vi "ApplicationStatusView.vi"(10 "Communicator":refnum<class "M1M3SAL.lvclass">, 11 "UserEvents":refnum<class "UserEvents.lvclass">) -> ()   [LabVIEW 2016, in "M1M3SupportViews.lvlib"]
uses:
  M1M3SupportViews.lvlib
  UserEvents/UserEvents.lvclass
  Communicator/M1M3SAL/M1M3SAL.lvclass
  DataTypes/Topics/Parts/SummaryStates.ctl
  DataTypes/Topics/Parts/DetailedStates.ctl
  UserEvents/UserEvents.lvclass/UserEvents.ctl
  DataTypes/Topics/M1M3SupportTopics.lvlib
panel:
  out "MinorRevision":u8[](array[numeric])
  out "MajorRevision":u8[](array[numeric])
  out "ReferencePosition":i32[](array[numeric])
  out "ILCUniqueId":i64[](array[numeric])
  out "SettingsApplied":string
  out "RecommendedSettingsVersion":string
  out "DetailedStates":T1
  out "ERxFrame":u32
  out "ETxFrame":u32
  out "FPGA Timestamp":dbl
  out "Timestamp":dbl
  out "SummaryStates":T2
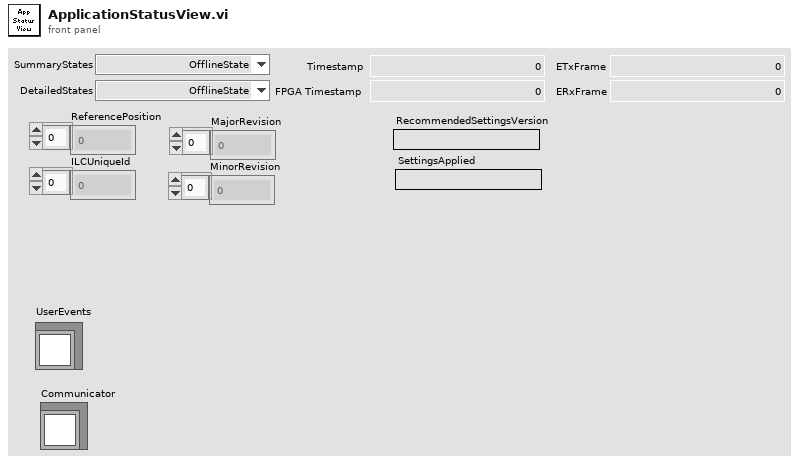
[diagram p1: front panel]
types:
  T1 = typedef "M1M3SupportTopics.lvlib/DetailedStates.ctl" = enum16{"OfflineState", "InitialState", "StandbyState", "DisabledState", "ParkedState", "FaultState", "ParkedMaintenanceState", "ActiveMaintenanceState"}
  T2 = typedef "M1M3SupportTopics.lvlib/SummaryStates.ctl" = enum16{"OfflineState", "StandbyState", "DisabledState", "EnabledState", "FaultState"}
  T3 = typedef "M1M3SupportTypes.lvlib/SummaryStates.ctl" = enum16{"OfflineState", "StandbyState", "DisabledState", "EnabledState", "FaultState"}
  T4 = typedef "M1M3SupportTopics.lvlib/Timestamp.ctl" = dbl
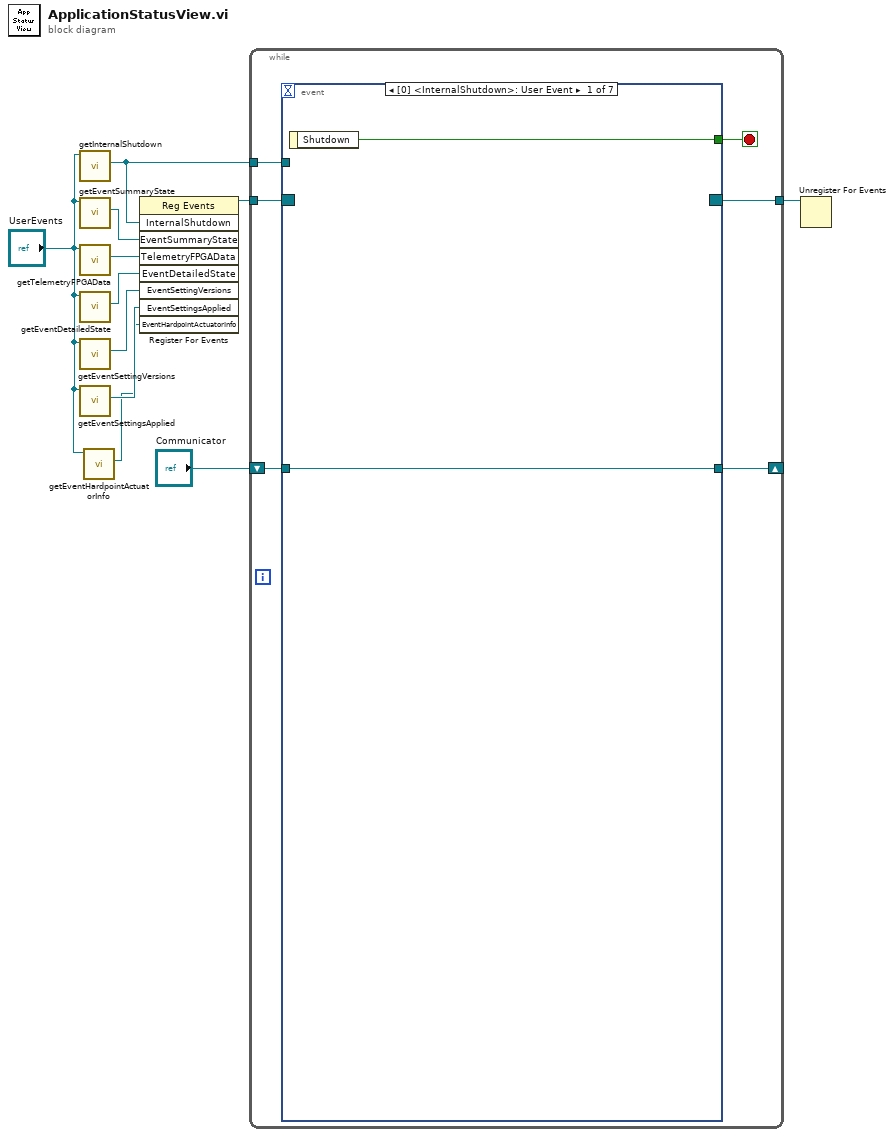
[diagram p0: block diagram]
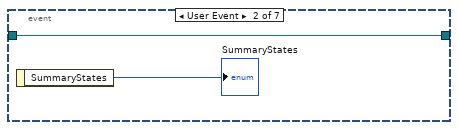
[diagram p2: hidden frame]
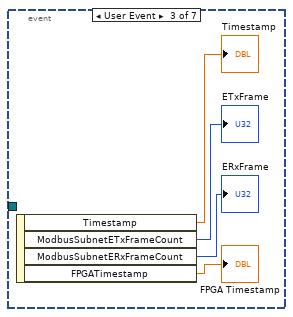
[diagram p3: hidden frame]
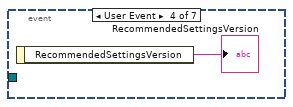
[diagram p4: hidden frame]
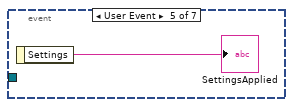
[diagram p5: hidden frame]
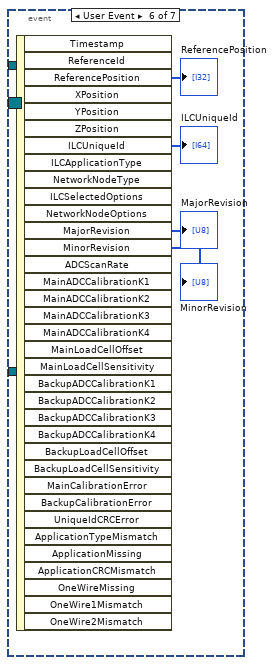
[diagram p6: hidden frame]
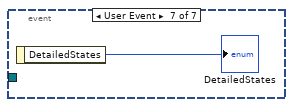
[diagram p7: hidden frame]
diagram:
  n1 = call "getInternalShutdown.vi"("UserEvents in"="UserEvents") -> ("InternalShutdown"=w7:refnum<user-event>)  [unwired: 9 in, 1 out]
  n2 = call "getEventSummaryState.vi"("UserEvents in"="UserEvents") -> ("EventSummaryState"=w11:refnum<user-event>)  [unwired: 9 in, 1 out]
  n3 = call "getTelemetryFPGAData.vi"("UserEvents in"="UserEvents") -> ("TelemetryFPGAData"=w6:refnum<user-event>)  [unwired: 9 in, 1 out]
  n4 = call "getEventDetailedState.vi"("UserEvents in"="UserEvents") -> ("EventDetailedState"=w5:refnum<user-event>)  [unwired: 9 in, 1 out]
  n5 = call "getEventSettingVersions.vi"("UserEvents in"="UserEvents") -> ("EventSettingVersions"=w4:refnum<user-event>)  [unwired: 9 in, 1 out]
  n6 = call "getEventSettingsApplied.vi"("UserEvents in"="UserEvents") -> ("EventSettingsApplied"=w3:refnum<user-event>)  [unwired: 9 in, 1 out]
  n7 = call "getEventHardpointActuatorInfo.vi"("UserEvents in"="UserEvents") -> ("EventHardpointActuatorInfo"=w1:refnum<user-event>)  [unwired: 9 in, 1 out]
  n8 = register-events(w7, w11, w6, w5, w4, w3, w1) -> (reference out=w10:refnum<event-registration>)  [unwired: 2 in, 1 out]
  n9 = while {
    tunnel: w10 -> [w17]
    tunnel: [w16] -> w9
    shift-right: [w13] -> _
    shift-left: "Communicator" -> [w14]
    tunnel: w7 -> [w12]
    stop <- w15 stop-if-true
    n10 = event shown="[0] <InternalShutdown>: User Event" {
      selector: w17 -> [_ _ _ _ _ _ _]
      dyn-events: [_ _ _ _ _ _ _] -> w16
      timeout: _ -> [_ _ _ _ _ _ _]
      tunnel: [w19 _ _ _ _ _ _] -> w15
      tunnel: w14 -> [w18 w21 _ _ _ _ _]
      tunnel: [w18 w21 _ _ _ _ _] -> w13
      tunnel: w12 -> [_ _ _ _ _ _ _]
      event User Event {
        n11 = event-data() -> ("Shutdown"=w19:bool)  [unwired: 1 in]
      }
      event User Event {
        n12 = event-data() -> ("SummaryStates"=→"SummaryStates":T3)  [unwired: 1 in]
      }
      event User Event {
        n13 = event-data() -> ("Timestamp"=→"Timestamp":T4, "ModbusSubnetETxFrameCount"=→"ETxFrame":u32, "ModbusSubnetERxFrameCount"=→"ERxFrame":u32, "FPGATimestamp"=→"FPGA Timestamp":dbl)  [unwired: 1 in]
      }
      event User Event {
        n14 = event-data() -> ("RecommendedSettingsVersion"=→"RecommendedSettingsVersion":string)  [unwired: 1 in]
      }
      event User Event {
        n15 = event-data() -> ("Settings"=→"SettingsApplied":string)  [unwired: 1 in]
      }
      event User Event {
        n16 = event-data() -> ("ReferencePosition"=→"ReferencePosition":i32[], "ILCUniqueId"=→"ILCUniqueId":i64[], "MajorRevision"=→"MajorRevision":u8[], "MinorRevision"=→"MinorRevision":u8[])  [unwired: 1 in, 31 out]
      }
      event User Event {
        n17 = event-data() -> ("DetailedStates"=→"DetailedStates":T1)  [unwired: 1 in]
      }
    }
  }
  n18 = Unregister For Events(event registration refnum=w9) -> ()  [unwired: 1 in, 1 out]
